vi "Build Run Parameters.vi"(8 "error in (no error)":errorcluster, 11 "CLI in":refnum<class "CLI.lvclass">) -> (0 "error out":errorcluster, 2 "Run Parameters":T1, 3 "CLI out":refnum<class "CLI.lvclass">)   [LabVIEW 2020, in "neg-pkg-cli.lvlib" / "CLI.lvclass"]
uses:
  CLI.lvclass
  build/ppl/neg-pkg.lvlibp/Action/Run Parameters.ctl
  build/ppl/neg-pkg.lvlibp/Status/Status.lvclass
  CLI.lvclass/CLI.ctl
  build/ppl/neg-pkg.lvlibp/Action/Action.lvclass
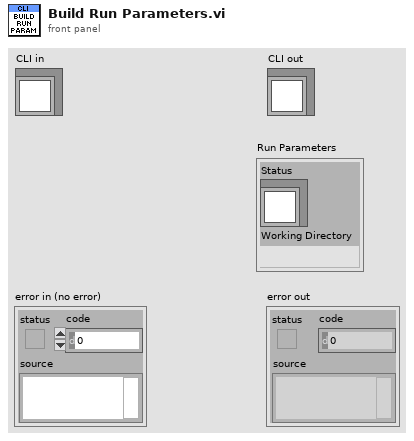
[diagram p1: front panel]
types:
  T1 = typedef "neg-pkg.lvlibp/Action.lvclass/Run Parameters.ctl" = cluster{"Status":refnum<class "Status.lvclass">, "Working Directory":path}
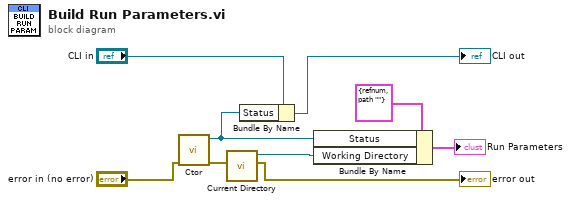
[diagram p0: block diagram]
diagram:
  n1 = call "Ctor.vi"("error in (no error)"="error in (no error)") -> ("error out"=w3:errorcluster, "Status out"=w5:refnum<class "Status.lvclass">)  [unwired: 9 in]
  n2 = call "Current Directory.vi"("error in (no error)"=w3) -> ("error out"=→"error out":errorcluster, "Current Directory"=w4:path)  [unwired: 9 in]
  n3 = Bundle By Name(cluster="CLI in", "Status"=w5) -> (→"CLI out":refnum<class "CLI.lvclass">)
  n4 = Bundle By Name(cluster=T1 {"Status"=refnum, "Working Directory"=path ""} ("Run Parameters"), "Status"=w5, "Working Directory"=w4) -> (→"Run Parameters":T1)
